vi "Create RotateFileHandler.vi"(4 "RotatorArgs":T1={"MaxSize_KB"=10000, "Compress"=FALSE, "MaxBackups"=5}, 6 "Flush Timeout_s (0 s)":dbl format="%#_13g", 7 "Formatter.lvclass":refnum<class "Formatter.lvclass">, 8 "error in":errorcluster, 9 "Level":T2, 10 "Name":string, 11 "Filepath":path) -> (0 "error out":errorcluster, 3 "FileHandler out":refnum<class "RotateFileHandler.lvclass">)   [LabVIEW 2024, in "RotateFileHandler.lvclass"]
doc: "Creates and initializes a new FileHandler object.\n\n____\nHAMPEL SOFTWARE ENGINEERING v2.2.2 (2025-01-16 15:41)"
uses:
  RotateFileHandler.lvclass
  <vilib>/Hampel Software Engineering/HSE Logger/LogLevel.ctl
  <vilib>/Hampel Software Engineering/HSE Logger/Formatter/Formatter.lvclass
  LogRotation/Args.ctl
  <vilib>/Hampel Software Engineering/HSE Logger/hse-logger.lvlib
  LogRotation/LogRotationHandler.lvclass
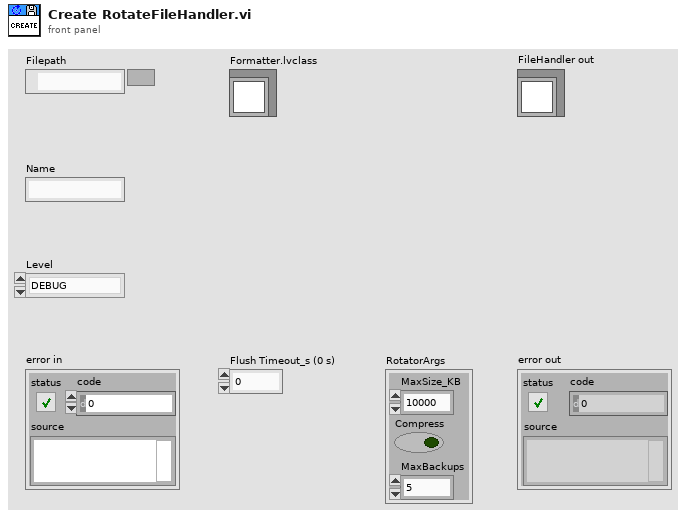
[diagram p1: front panel]
types:
  T1 = typedef "LogRotationHandler.lvclass/Args.ctl" = cluster{"MaxSize_KB":i32, "Compress":bool, "MaxBackups":i32}
  T2 = typedef "hse-logger.lvlib/LogLevel.ctl" = enum16{"DEBUG", "INFO", "WARNING", "ERROR", "CRITICAL"}
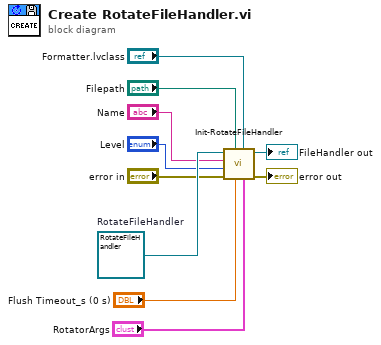
[diagram p0: block diagram]
diagram:
  w10 = refnum<class "RotateFileHandler.lvclass"> refnum  # RotateFileHandler
  n1 = call "Init-RotateFileHandler.vi"("RotatorArgs"="RotatorArgs", "Formatter.lvclass"="Formatter.lvclass", "Flush Timeout_s (5 s)"="Flush Timeout_s (0 s)", "Filepath"="Filepath", "error in (no error)"="error in", "Level"="Level", "Name"="Name", "FileHandler in"=w10) -> ("error out"=→"error out":errorcluster, "FileHandler out"=→"FileHandler out":refnum<class "RotateFileHandler.lvclass">)  [unwired: 2 in]
